vi "Analyze Data.vi"(8 "error in":errorcluster, 11 "CRDS in":refnum<class "CRDS.lvclass">) -> (0 "error out":errorcluster, 3 "CRDS out":refnum<class "CRDS.lvclass">)   [LabVIEW 2015, in "CRDS Lib.lvlib" / "CRDS.lvclass"]
doc: "Analyze Data takes the stored ringdown data (1000 shots per cell) and:\n1) Calculates the ringdown decay constant tau\n2) Averages tau0 data as necessary\n3) Corrects the tau data for Rayleigh scattering\n4) Stores a 1-D array of taus returned on a 1 kHz basis (8k taus) if a jump drive (U:) is connected\n5) Flattens the data into a string and stuffs the string into the <b>data</b> shared variable for display on the UI.\n\nThis VI will not be called if the data is not \"good\" (that is, if an error was thrown in the <B>Get Data</B> routine. If an error is thrown while the data is being retrieved, then the data will not be sent to the UI."
uses:
  CRDS.lvclass
  Instrument/Instrument.lvclass/Instrument.ctl
  CRDS.lvclass/CRDS.ctl
  Data/Main/CRDS Data.lvclass
  Cell/CRDS Cell.lvclass/CRDS Cell.ctl
  Data/Cell/CRDS Cell Data.lvclass/CRDS Cell Data.ctl
  Cell/Read Laser Data.vi
  Data/Cell/Write Laser Data.vi
  Instrument/Write Data.vi
  Read Saving RDs.vi
  Read Cells.vi
  Data/Main/Read filter.vi
  Write Cells.vi
  Data/Data.lvclass
  Cell/CRDS Cell.lvclass
  Data/Cell/CRDS Cell Data.lvclass
  Instrument/Instrument.lvclass
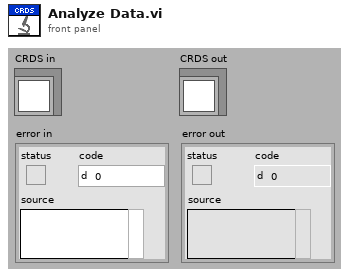
[diagram p1: front panel]
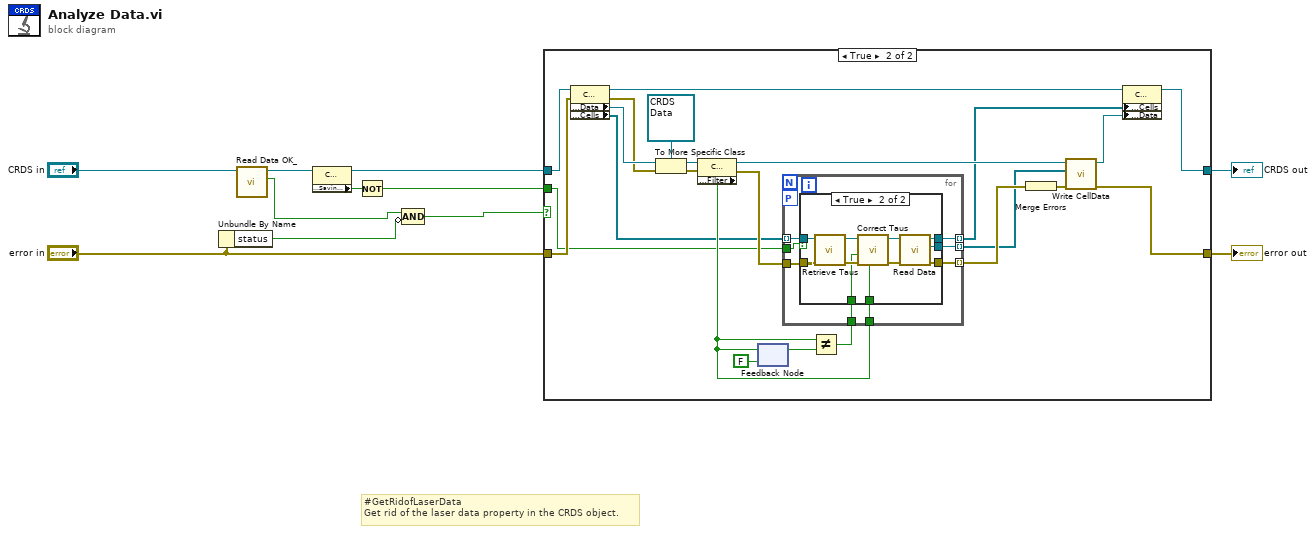
[diagram p0: block diagram]
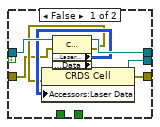
[diagram p3: hidden frame]
diagram:
  # "#GetRidofLaserData\nGet rid of the laser data property in the CRDS object."
  n1 = Unbundle By Name("error in") -> ("status"=w3:bool)
  n2 = call "Read Data OK_.vi"("Instrument in"="CRDS in") -> ("Data OK?"=w4:bool, "Instrument out"=w7:refnum<class "CRDS.lvclass">)  [unwired: 8 in, 1 out]
  n3 = property class="CRDS"(reference=w7) -> (reference out=w6:refnum<class "CRDS.lvclass">, "Data Access:Saving RDs"=w5:bool)  [unwired: 1 in, 1 out]
  n4 = Not(x=w5) -> (.not. x?=w1:bool)
  n5 = Compound Arithmetic op=AND(w4, invert w3) -> (w2:bool)
  n6 = case shown="True" w2 {
    tunnel: w6 -> [w13 w35]
    tunnel: "error in" -> [w12 w16]
    tunnel: [w13 w33] -> w10
    tunnel: [w12 w36] -> w9
    tunnel: w1 -> [_ w14]
    frame False {
    }
    frame True {
      n7 = property class="CRDS"(reference=w35, error in=w16) -> (reference out=w19:refnum<class "CRDS.lvclass">, error out=w15:errorcluster, "Accessors:Data"=w23:refnum<class "Data.lvclass">, "Data Access:Cells"=w17:refnum<class "CRDS Cell.lvclass">[])
      n8 = To More Specific Class(target class=refnum<class "CRDS Data.lvclass"> refnum ("reference out"), reference=w23, error in=w15) -> (specific class reference=w22:refnum<class "CRDS Data.lvclass">, error out=w18:errorcluster)
      n9 = property class="CRDS"(reference=w22, error in=w18) -> (reference out=w24:refnum<class "CRDS Data.lvclass">, error out=w26:errorcluster, "Accessors:Filter"=w27:bool)
      n10 = feedback #1(FALSE ("filter")) -> (w30:bool)
      n11 = feedback-in #1(w27) -> ()
      n12 = Not Equal?(x=w27, y=w30) -> (x != y?=w28:bool)
      n13 = for "Initial extinction calculation" {
        tunnel: w17 -> [w43] mode=indexing
        tunnel: w26 -> [w38]
        tunnel: w27 -> [w44]
        tunnel: [w42] -> w21 mode=indexing
        tunnel: [w41] -> w32 mode=indexing
        tunnel: [w40] -> w31 mode=indexing
        tunnel: w28 -> [w39]
        workers-P: _ -> [_]
        tunnel: w14 -> [w37]
        n14 = case shown="True" w37 {
          tunnel: w44 -> [_ w63]
          tunnel: w43 -> [w52 w60]
          tunnel: [w50 w57] -> w42
          tunnel: [w51 w56] -> w41
          tunnel: [w48 w55] -> w40
          tunnel: w39 -> [_ w54]
          tunnel: w38 -> [w45 w53]
          frame False {
            n15 = property class="CRDS Cell"(reference=w52, error in=w45) -> (reference out=w50:refnum<class "CRDS Cell.lvclass">, error out=w46:errorcluster, "Accessors:Laser Data"=w47:i16[][], "Accessors:Data"=w49:refnum<class "CRDS Cell Data.lvclass">)
            n16 = property class="CRDS Cell"(reference=w49, error in=w46, "Accessors:Laser Data"=w47) -> (reference out=w48:refnum<class "CRDS Cell Data.lvclass">, error out=w51:errorcluster)
          }
          frame True {
            n17 = call "Retrieve Taus.vi"("error in"=w53, "CRDS Cell in"=w60) -> ("error out"=w61:errorcluster, "CRDS Cell out"=w62:refnum<class "CRDS Cell.lvclass">)  [unwired: 7 in, 1 out]
            n18 = call "Correct Taus.vi"("Filter?"=w63, "error in"=w61, "filter changed?"=w54, "CRDS Cell in"=w62) -> ("error out"=w58:errorcluster, "CRDS Cell out"=w59:refnum<class "CRDS Cell.lvclass">)  [unwired: 6 in]
            n19 = call "Read Data.vi"("error in"=w58, "CRDS Cell in"=w59) -> ("error out"=w56:errorcluster, "CRDS Cell"=w55:refnum<class "CRDS Cell Data.lvclass">, "CRDS Cell out"=w57:refnum<class "CRDS Cell.lvclass">)  [unwired: 7 in]
          }
        }
      }
      n20 = Merge Errors(w32) -> (w25:errorcluster)
      n21 = call "Write CellData.vi"("error in"=w25, "CellData"=w31, "CRDS Data in"=w24) -> ("error out"=w36:errorcluster, "CRDS Data out"=w20:refnum<class "CRDS Data.lvclass">)  [unwired: 7 in]
      n22 = property class="CRDS"(reference=w19, "Data Access:Cells"=w21, "Accessors:Data"=w20) -> (reference out=w33:refnum<class "CRDS.lvclass">)  [unwired: 1 in, 1 out]
    }
  }
  "error out" <- w9
  "CRDS out" <- w10
